vi "Rx Buffered Packet Page.vi"(8 "error in (no error)":errorcluster, 11 "Node Ptr":T4 format="%.0x") -> (0 "error out":errorcluster)   [LabVIEW 2016, in "UDP-Custom-Device System Explorer.lvlib"]
uses:
  UDP-Custom-Device System Explorer.lvlib
  Shared/Types/Shared - New Data Options.ctl
  Shared/Types/Shared - Receive Buffer Options.ctl
  Shared/Types/Shared - Pointer Encoding.ctl
  <vilib>/NI Veristand/Custom Device API/Custom Device Item Ref.ctl
  Types/Page References/Refs - Rx Buffered Data Packet Page.ctl
  <vilib>/NI VeriStand/Custom Device API/Custom Device API.lvlib
  Property Accessors/Shared Packet Accessors.lvlib
  Property Accessors/Buffered Data Packet.lvlib
  Property Accessors/Rx Packet Accessors.lvlib
  Shared/UDP-Custom-Device Shared.lvlib
panel:
  in  "Debug Mode":bool caption="Auto-Assign Local NIC"
  in  "Buffer Options":T1
  in  "New Data Options":T2
  in  "Pointer Encoding":T3
  in  "Multicast?":bool caption="Auto-Assign Local NIC"
  in  "Multicast IP Address":string
  in  "Read Timeout (ms)":i32
  in  "Prepend\nHeader?":bool caption="Auto-Assign Local NIC"
  in  "External Buffer?":bool
  in  "Buffer Size (bytes)":u32
  in  "Configure Header":bool
  in  "Endianness":u16(ring) items=["big-endian"=0, "little-endian"=2]
  in  "General Header 3":cluster{"Section Name":string}={"Section Name"="Network Settings"}
  out "Packet ID":i32
  in  "Auto-Assign Local NIC":bool
  in  "Port":u16
  in  "IP Address of Local NIC":string
  in  "Description":string
  in  "Name":string
  in  "General Header 2":cluster{"Section Name":string}={"Section Name"="Buffer Configuration"}
  in  "SHDocVw.IWebBrowser":refnum<k7>(container)
  in  "General Header":cluster{"Section Name":string}={"Section Name"="Packet Configuration"}
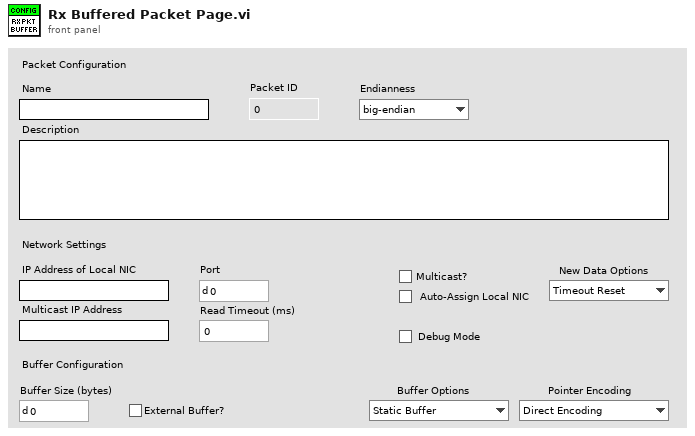
[diagram p1: front panel]
types:
  T1 = typedef "UDP-Custom-Device Shared.lvlib/Shared - Receive Buffer Options.ctl" = enum16{"Static Buffer", "Circular Buffer", "Circular Buffer + Size"}
  T2 = typedef "UDP-Custom-Device Shared.lvlib/Shared - New Data Options.ctl" = enum16{"Timeout Reset", "Counter"}
  T3 = typedef "UDP-Custom-Device Shared.lvlib/Shared - Pointer Encoding.ctl" = enum16{"Direct Encoding", "Conversion Encoding"}
  T4 = typedef "Custom Device API.lvlib/Custom Device Item Ref.ctl" = u64
  T5 = typedef "UDP-Custom-Device System Explorer.lvlib/Refs - Rx Buffered Data Packet Page.ctl" = cluster{"Name":refnum<vi>, "Description":refnum<vi>, "Packet ID":refnum<vi>, "Endianness":refnum<vi>, "Prepend\nHeader?":refnum<vi>, "Configure Header":refnum<vi>, "IP Address of Local NIC":refnum<vi>, "Port":refnum<vi>, "Auto-Assign Local NIC":refnum<vi>, "External Buffer?":refnum<vi>, "Buffer Size (bytes)":refnum<vi>, "Read Timeout (ms)":refnum<vi>, "Multicast?":refnum<vi>, "Multicast IP Address":refnum<vi>, "Pointer Encoding":refnum<vi>, "New Data Options":refnum<vi>, "Debug Mode":refnum<vi>, "Buffer Options":refnum<vi>}
  T6 = enum8{"Enabled", "Disabled", "Disabled and Grayed Out"}
  T7 = typedef "Custom Device API.lvlib/Custom Device Commands.ctl" = enum16{"Default", "Item renamed", "Shutdown", "Dynamic button pressed"}
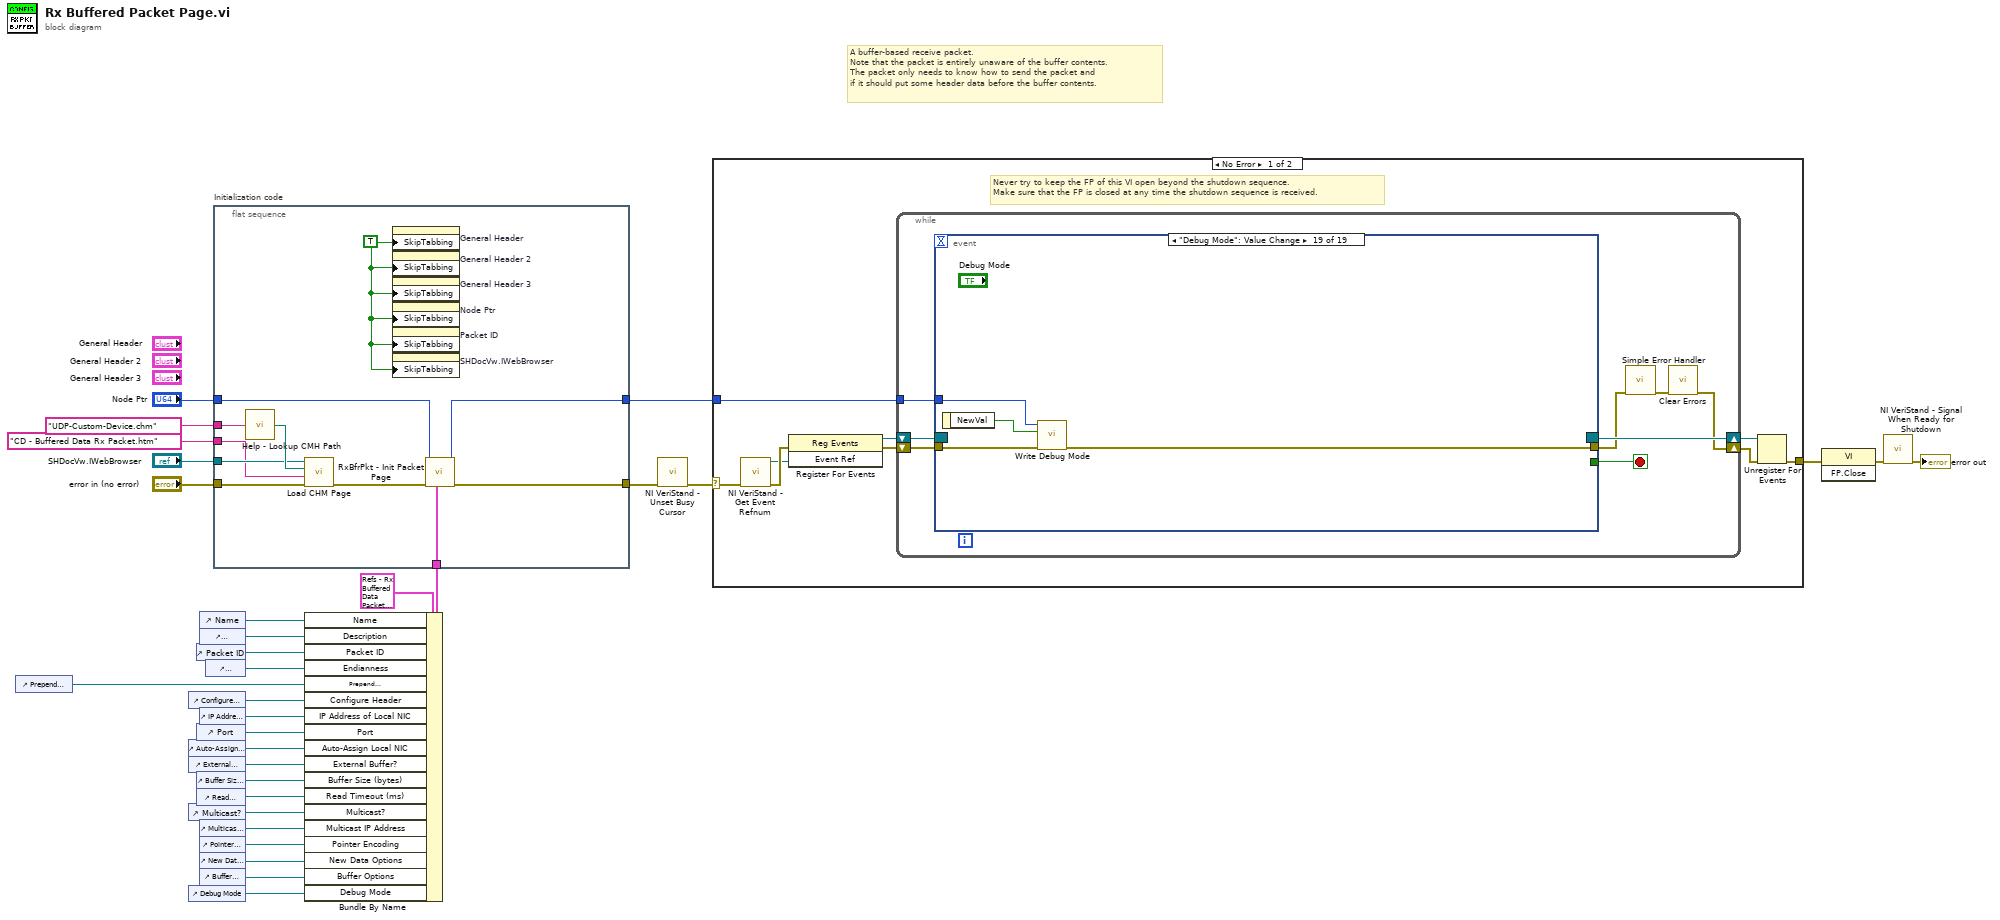
[diagram p0: block diagram]
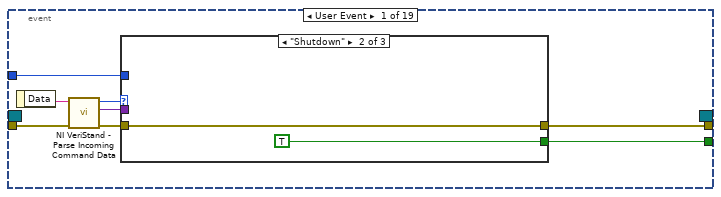
[diagram p2: hidden frame]
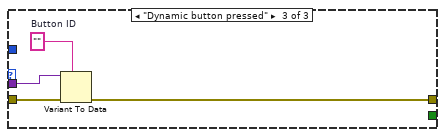
[diagram p4: hidden frame]
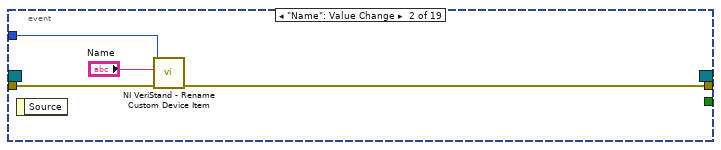
[diagram p5: hidden frame]
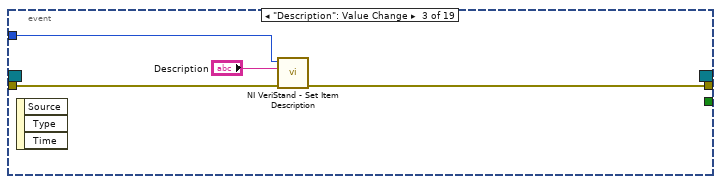
[diagram p6: hidden frame]
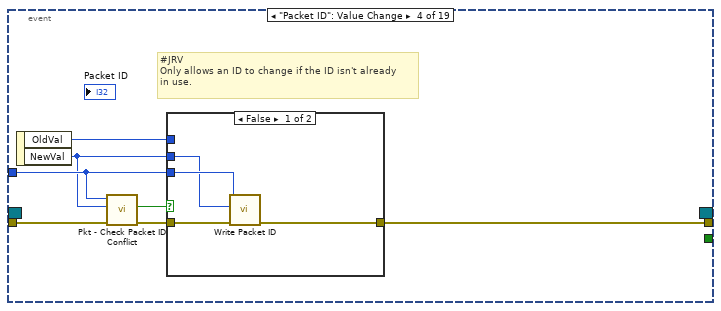
[diagram p7: hidden frame]
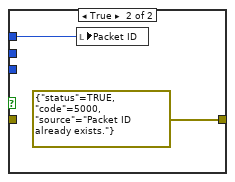
[diagram p8: hidden frame]
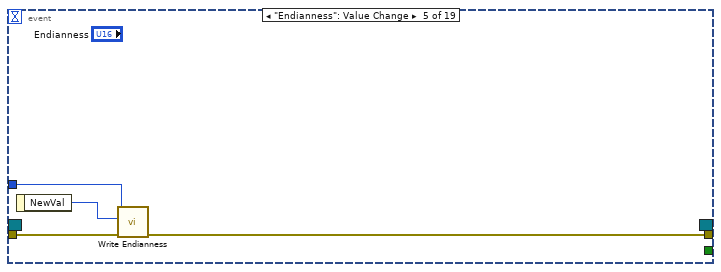
[diagram p9: hidden frame]
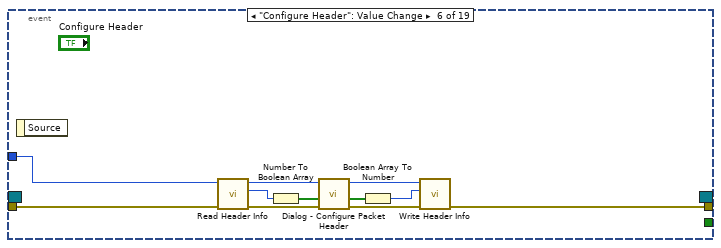
[diagram p10: hidden frame]
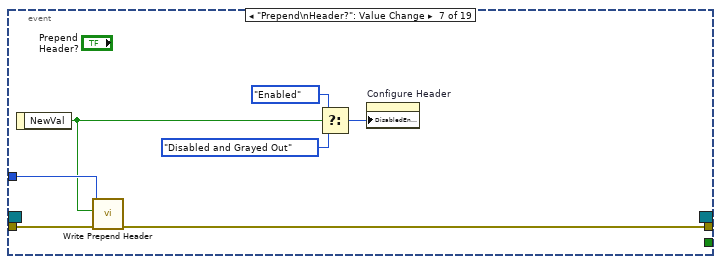
[diagram p11: hidden frame]
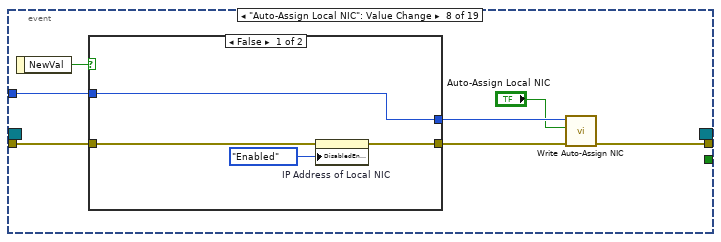
[diagram p12: hidden frame]
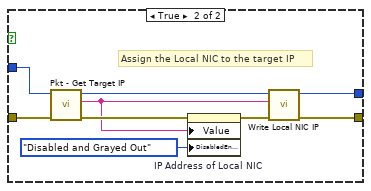
[diagram p13: hidden frame]
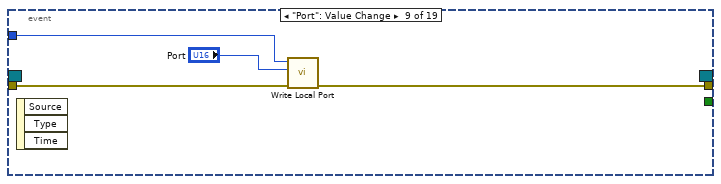
[diagram p14: hidden frame]
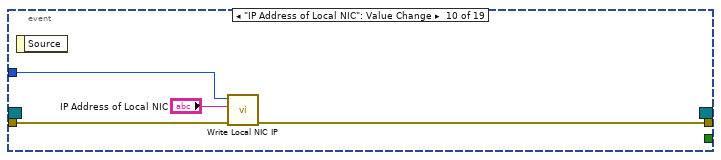
[diagram p15: hidden frame]
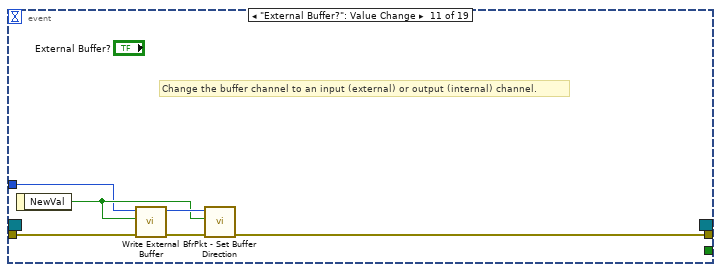
[diagram p16: hidden frame]
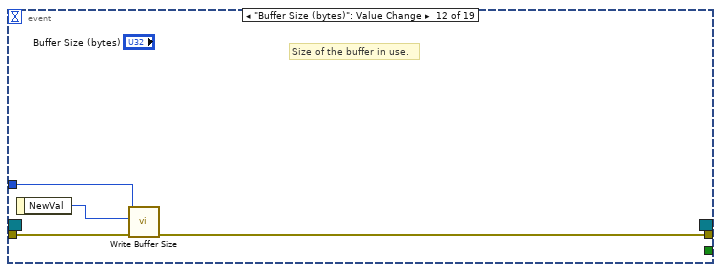
[diagram p17: hidden frame]
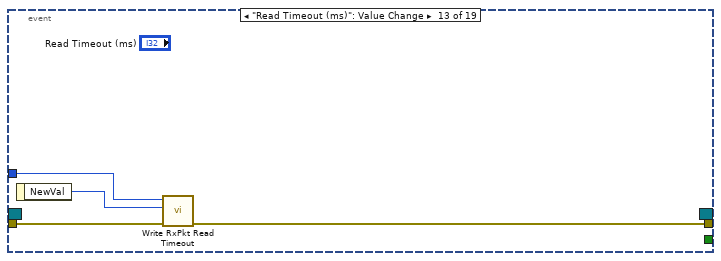
[diagram p18: hidden frame]
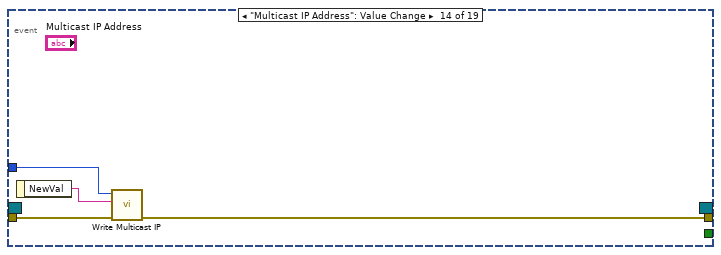
[diagram p19: hidden frame]
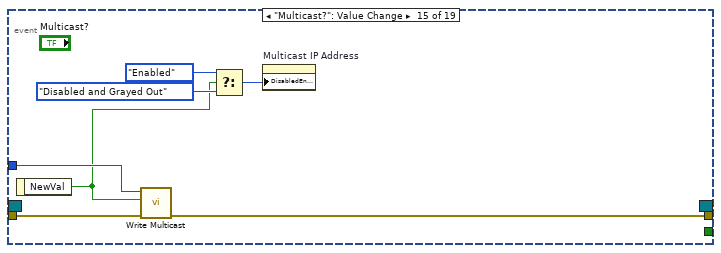
[diagram p20: hidden frame]
diagram:
  # "A buffer-based receive packet.\nNote that the packet is entirely unaware of the buffer contents.\nThe packet only needs to know how to send the packet and\nif it should put some header data before the buffer contents."
  n1 = control-ref of="Prepend\nHeader?"() -> (w14:refnum<vi>)
  n2 = control-ref of="Configure Header"() -> (w13:refnum<vi>)
  n3 = control-ref of="Auto-Assign Local NIC"() -> (w10:refnum<vi>)
  n4 = control-ref of="External Buffer?"() -> (w9:refnum<vi>)
  n5 = control-ref of="Multicast?"() -> (w6:refnum<vi>)
  n6 = control-ref of="Debug Mode"() -> (w2:refnum<vi>)
  n7 = control-ref of="Packet ID"() -> (w16:refnum<vi>)
  n8 = control-ref of="Port"() -> (w11:refnum<vi>)
  n9 = control-ref of="Buffer Size (bytes)"() -> (w8:refnum<vi>)
  n10 = control-ref of="Read Timeout (ms)"() -> (w7:refnum<vi>)
  n11 = control-ref of="Name"() -> (w18:refnum<vi>)
  n12 = control-ref of="Description"() -> (w17:refnum<vi>)
  n13 = control-ref of="IP Address of Local NIC"() -> (w12:refnum<vi>)
  n14 = control-ref of="Multicast IP Address"() -> (w5:refnum<vi>)
  n15 = control-ref of="Pointer Encoding"() -> (w4:refnum<vi>)
  n16 = control-ref of="New Data Options"() -> (w3:refnum<vi>)
  n17 = control-ref of="Buffer Options"() -> (w1:refnum<vi>)
  n18 = control-ref of="Endianness"() -> (w15:refnum<vi>)
  n19 = flat-sequence "Initialization code" {
    tunnel: "error in (no error)" -> [w41]
    tunnel: "Node Ptr" -> [w36]
    tunnel: [w33] -> w27
    tunnel: "SHDocVw.IWebBrowser" -> [w39]
    tunnel: "CD - Buffered Data Rx Packet.htm" ("CD_CHM_Section") -> [w38]
    tunnel: "UDP-Custom-Device.chm" ("CD_CHM_FileName") -> [w40]
    tunnel: [w35] -> w22
    tunnel: w19 -> [w32]
    frame #0 {
      w37 = TRUE ("Skip When Tabbing")
      n20 = call "Help - Lookup CMH Path.vi"("Main CMH File"=w40) -> ("Compiled CMH Path"=w42:path)
      n21 = call <vilib>:"Load CHM Page.vi"("error in (no error)"=w41, "HTML File"=w38, "Compiled CHM Path"=w42, "Web Browser Reference"=w39) -> ("error out"=w34:errorcluster)  [unwired: 7 in]
      n22 = property on="General Header" class="Clust (strict)"("SkipTabbing"=w37) -> ()  [unwired: 2 in, 2 out]
      n23 = property on="General Header 2" class="Clust (strict)"("SkipTabbing"=w37) -> ()  [unwired: 2 in, 2 out]
      n24 = property on="General Header 3" class="Clust (strict)"("SkipTabbing"=w37) -> ()  [unwired: 2 in, 2 out]
      n25 = property on="Node Ptr" class="DigNum (strict)"("SkipTabbing"=w37) -> ()  [unwired: 2 in, 2 out]
      n26 = property on="Packet ID" class="DigNum (strict)"("SkipTabbing"=w37) -> ()  [unwired: 2 in, 2 out]
      n27 = property on="SHDocVw.IWebBrowser" class="AXCont"("SkipTabbing"=w37) -> ()  [unwired: 2 in, 2 out]
      n28 = call "RxBfrPkt - Init Packet Page.vi"("Rx Buffered Data Packet Refs"=w32, "error in (no error)"=w34, "Node Ptr In"=w36) -> ("error out"=w33:errorcluster, "Node Ptr Out"=w35:T4)  [unwired: 7 in]
    }
  }
  n29 = Bundle By Name(cluster=T5 {"Name"=refnum, "Description"=refnum, "Packet ID"=refnum, "Endianness"=refnum, "Prepend\nHeader?"=refnum, "Configure Header"=refnum, "IP Address of Local NIC"=refnum, "Port"=refnum, "Auto-Assign Local NIC"=refnum, "External Buffer?"=refnum, "Buffer Size (bytes)"=refnum, "Read Timeout (ms)"=refnum, "Multicast?"=refnum, "Multicast IP Address"=refnum, "Pointer Encoding"=refnum, "New Data Options"=refnum, "Debug Mode"=refnum, "Buffer Options"=refnum} ("Rx Buffered Data Packet Refs"), "Name"=w18, "Description"=w17, "Packet ID"=w16, "Endianness"=w15, "Prepend\nHeader?"=w14, "Configure Header"=w13, "IP Address of Local NIC"=w12, "Port"=w11, "Auto-Assign Local NIC"=w10, "External Buffer?"=w9, "Buffer Size (bytes)"=w8, "Read Timeout (ms)"=w7, "Multicast?"=w6, "Multicast IP Address"=w5, "Pointer Encoding"=w4, "New Data Options"=w3, "Buffer Options"=w1, "Debug Mode"=w2) -> (w19:T5)
  n30 = call <vilib>:"NI VeriStand - Unset Busy Cursor.vi"("error in (no error)"=w27) -> ("error out"=w26:errorcluster)  [unwired: 10 out]
  n31 = case shown="No Error" w26 {
    selector: w26 -> [w43 w189]
    tunnel: [w48 w187] -> w31
    tunnel: w22 -> [w44 _]
    frame No Error {
      # "Never try to keep the FP of this VI open beyond the shutdown sequence.\nMake sure that the FP is closed at any time the shutdown sequence is received."
      n32 = call <vilib>:"NI VeriStand - Get Event Refnum.vi"("error in (no error)"=w43) -> ("error out"=w51:errorcluster, "Event Ref"=w47:refnum<user-event>)  [unwired: 9 out]
      n33 = register-events(error in=w51, w47) -> (reference out=w45:refnum<event-registration>, error out=w46:errorcluster)  [unwired: 1 in]
      n34 = while {
        tunnel: w44 -> [w55]
        shift-right: [w52] -> w49
        shift-left: w46 -> [w58]
        shift-right: [w59] -> w50
        shift-left: w45 -> [w57]
        stop <- w56 stop-if-true
        n35 = event shown="[18] \"Debug Mode\": Value Change" {
          selector: w57 -> [_ _ _ _ _ _ _ _ _ _ _ _ _ _ _ _ _ _ _]
          dyn-events: [_ _ _ _ _ _ _ _ _ _ _ _ _ _ _ _ _ _ _] -> w59
          timeout: _ -> [_ _ _ _ _ _ _ _ _ _ _ _ _ _ _ _ _ _ _]
          tunnel: w58 -> [w67 w78 w82 w87 w98 w107 w114 w124 w140 w145 w147 w153 w157 w161 w169 w173 w176 w182 w184]
          tunnel: [w63 _ _ _ _ _ _ _ _ _ _ _ _ _ _ _ _ _ _] -> w56
          tunnel: [w62 w76 w79 w89 w97 w101 w111 w119 w139 w144 w146 w152 w156 w160 w168 w171 w175 w179 w183] -> w54
          tunnel: w55 -> [w61 w77 w81 w88 w99 w108 w115 w123 w141 w142 w148 w155 w159 w163 w170 w174 w178 w181 w186]
          event User Event {
            n36 = event-data() -> ("Data"=w66:string)  [unwired: 1 out]
            n37 = call <vilib>:"NI VeriStand - Parse Incoming Command Data.vi"("error in (no error)"=w67, "Incoming data"=w66) -> ("error out"=w65:errorcluster, "Outgoing data"=w60:variant, "Action"=w64:T7)  [unwired: 7 out]
            n38 = case shown="\"Shutdown\"" w64 {
              tunnel: w65 -> [w68 w69 w74]
              tunnel: [_ TRUE _] -> w63
              tunnel: [w68 w69 w71] -> w62
              tunnel: w61 -> [_ _ _]
              tunnel: w60 -> [_ _ w73]
              frame "Default", Default {
              }
              frame "Shutdown" {
              }
              frame "Dynamic button pressed" {
                w72 = ""  # Button ID
                n39 = Variant To Data(error in=w74, type=w72, Variant=w73) -> (error out=w71:errorcluster)  [unwired: 1 out]
              }
            }
          }
          event "Name": Value Change {
            n40 = event-data() -> ()  [unwired: 2 out]
            n41 = call <vilib>:"NI VeriStand - Rename Custom Device Item.vi"("error in (no error)"=w78, "New Name"="Name", "Item Ref in"=w77) -> ("error out"=w76:errorcluster)  [unwired: 6 in, 2 out]
          }
          event "Description": Value Change {
            n42 = event-data() -> ()  [unwired: 4 out]
            n43 = call <vilib>:"NI VeriStand - Set Item Description.vi"("error in (no error)"=w82, "Description"="Description", "Item Ref in"=w81) -> ("error out"=w79:errorcluster)  [unwired: 6 in, 2 out]
          }
          event "Packet ID": Value Change {
            # "#JRV\nOnly allows an ID to change if the ID isn't already\nin use."
            n44 = event-data() -> ("OldVal"=w83:i32, "NewVal"=w84:i32)  [unwired: 1 out]
            n45 = call "Pkt - Check Packet ID Conflict.vi"("error in (no error)"=w87, "New ID"=w84, "Packet Ref In"=w88) -> ("error out"=w86:errorcluster, "Conflicting ID?"=w85:bool)  [unwired: 7 in]
            n46 = case shown="False" w85 {
              tunnel: [w92 errorcluster {"status"=TRUE, "code"=5000, "source"="Packet ID already exists."} ("error out")] -> w89
              tunnel: w88 -> [w91 _]
              tunnel: w86 -> [w93 _]
              tunnel: w84 -> [w90 _]
              tunnel: w83 -> [_ w95]
              frame False {
                n47 = call "Write Packet ID.vi"("error in (no error)"=w93, "Packet ID"=w90, "Node Ptr"=w91) -> ("error out"=w92:errorcluster)  [unwired: 7 in, 1 out]
              }
              frame True {
                n48 = local write "Packet ID"(w95) -> ()
              }
            }
          }
          event "Endianness": Value Change {
            n49 = event-data() -> ("NewVal"=w96:u16)  [unwired: 1 out]
            n50 = call "Write Endianness.vi"("error in (no error)"=w98, "Endianness"=w96, "Node Ptr"=w99) -> ("error out"=w97:errorcluster)  [unwired: 7 in, 1 out]
          }
          event "Configure Header": Value Change {
            n51 = event-data() -> ()  [unwired: 2 out]
            n52 = call "Read Header Info.vi"("error in (no error)"=w107, "Node Ptr"=w108) -> ("error out"=w106:errorcluster, "Header Info"=w105:u32, "Node Ptr out"=w104:T4)  [unwired: 7 in]
            n53 = Number To Boolean Array(number=w105) -> (Boolean array=w110:bool[])
            n54 = call "Dialog - Configure Packet Header.vi"("error in (no error)"=w106, "Header Elements In"=w110, "Packet Ref in"=w104) -> ("error out"=w102:errorcluster, "Header Elements Out"=w109:bool[], "Packet Ref out"=w103:T4)  [unwired: 6 in]
            n55 = Boolean Array To Number(Boolean array=w109) -> (number=w100:u32)
            n56 = call "Write Header Info.vi"("error in (no error)"=w102, "Header Info"=w100, "Node Ptr"=w103) -> ("error out"=w101:errorcluster)  [unwired: 7 in, 1 out]
          }
          event "Prepend\nHeader?": Value Change {
            n57 = event-data() -> ("NewVal"=w113:bool)  [unwired: 1 out]
            n58 = call "Write Prepend Header.vi"("error in (no error)"=w114, "Prepend Header"=w113, "Node Ptr"=w115) -> ("error out"=w111:errorcluster)  [unwired: 7 in, 1 out]
            n59 = Select(t=T6."Enabled" ("Disabled"), s=w113, f=T6."Disabled and Grayed Out" ("Disabled")) -> (s? t:f=w112:T6)
            n60 = property on="Configure Header" class="Bool"("DisabledEnum"=w112) -> ()  [unwired: 2 in, 2 out]
          }
          event "Auto-Assign Local NIC": Value Change {
            n61 = event-data() -> ("NewVal"=w122:bool)  [unwired: 1 out]
            n62 = case shown="False" w122 {
              tunnel: w123 -> [w126 w136]
              tunnel: w124 -> [w127 w137]
              tunnel: [w128 w129] -> w120
              tunnel: [w126 w132] -> w121
              frame False {
                n63 = property on="IP Address of Local NIC" class="Str"(error in=w127, "DisabledEnum"=T6."Enabled" ("Disabled")) -> (error out=w128:errorcluster)  [unwired: 1 in, 1 out]
              }
              frame True {
                # "Assign the Local NIC to the target IP"
                n64 = call "Pkt - Get Target IP.vi"("error in"=w137, "Item Ref in"=w136) -> ("error out"=w135:errorcluster, "IPAddress"=w131:string, "Item Ref out"=w133:T4)  [unwired: 7 in]
                n65 = property on="IP Address of Local NIC" class="Str"(error in=w135, "Value"=w131, "DisabledEnum"=T6."Disabled and Grayed Out" ("Disabled")) -> (error out=w130:errorcluster)  [unwired: 1 in, 1 out]
                n66 = call "Write Local NIC IP.vi"("error in (no error)"=w130, "IP Address of Local NIC"=w131, "Node Ptr"=w133) -> ("error out"=w129:errorcluster, "Node Ptr out"=w132:T4)  [unwired: 7 in]
              }
            }
            n67 = call "Write Auto-Assign NIC.vi"("error in (no error)"=w120, "Auto-Assign NIC"="Auto-Assign Local NIC", "Node Ptr"=w121) -> ("error out"=w119:errorcluster)  [unwired: 7 in, 1 out]
          }
          event "Port": Value Change {
            n68 = event-data() -> ()  [unwired: 4 out]
            n69 = call "Write Local Port.vi"("error in (no error)"=w140, "Port"="Port", "Node Ptr"=w141) -> ("error out"=w139:errorcluster)  [unwired: 7 in, 1 out]
          }
          event "IP Address of Local NIC": Value Change {
            n70 = event-data() -> ()  [unwired: 2 out]
            n71 = call "Write Local NIC IP.vi"("error in (no error)"=w145, "IP Address of Local NIC"="IP Address of Local NIC", "Node Ptr"=w142) -> ("error out"=w144:errorcluster)  [unwired: 7 in, 1 out]
          }
          event "External Buffer?": Value Change {
            # "Change the buffer channel to an input (external) or output (internal) channel."
            n72 = event-data() -> ("NewVal"=w149:bool)  [unwired: 1 out]
            n73 = call "Write External Buffer.vi"("error in (no error)"=w147, "External Buffer"=w149, "Node Ptr"=w148) -> ("error out"=w151:errorcluster, "Node Ptr out"=w150:T4)  [unwired: 7 in]
            n74 = call "BfrPkt - Set Buffer Direction.vi"("error in (no error)"=w151, "External?"=w149, "Node Ptr"=w150) -> ("error out"=w146:errorcluster)  [unwired: 7 in, 1 out]
          }
          event "Buffer Size (bytes)": Value Change {
            # "Size of the buffer in use."
            n75 = event-data() -> ("NewVal"=w154:u32)  [unwired: 1 out]
            n76 = call "Write Buffer Size.vi"("error in (no error)"=w153, "Buffer Size"=w154, "Node Ptr"=w155) -> ("error out"=w152:errorcluster)  [unwired: 7 in, 1 out]
          }
          event "Read Timeout (ms)": Value Change {
            n77 = event-data() -> ("NewVal"=w158:i32)  [unwired: 1 out]
            n78 = call "Write RxPkt Read Timeout.vi"("error in (no error)"=w157, "Read Timeout"=w158, "Node Ptr"=w159) -> ("error out"=w156:errorcluster)  [unwired: 7 in, 1 out]
          }
          event "Multicast IP Address": Value Change {
            n79 = event-data() -> ("NewVal"=w162:string)  [unwired: 1 out]
            n80 = call "Write Multicast IP.vi"("error in (no error)"=w161, "Multicast IP Address"=w162, "Node Ptr"=w163) -> ("error out"=w160:errorcluster)  [unwired: 7 in, 1 out]
          }
          event "Multicast?": Value Change {
            n81 = event-data() -> ("NewVal"=w165:bool)  [unwired: 1 out]
            n82 = call "Write Multicast.vi"("error in (no error)"=w169, "Multicast"=w165, "Node Ptr"=w170) -> ("error out"=w168:errorcluster)  [unwired: 7 in, 1 out]
            n83 = Select(t=T6."Enabled" ("Disabled"), s=w165, f=T6."Disabled and Grayed Out" ("Disabled")) -> (s? t:f=w164:T6)
            n84 = property on="Multicast IP Address" class="Str"("DisabledEnum"=w164) -> ()  [unwired: 2 in, 2 out]
          }
          event Value Change {
            n85 = event-data() -> ("NewVal"=w172:T3)  [unwired: 1 out]
            n86 = call "Write Pointer Encoding.vi"("error in (no error)"=w173, "Pointer Encoding"=w172, "Node Ptr"=w174) -> ("error out"=w171:errorcluster)  [unwired: 7 in, 1 out]
          }
          event Value Change {
            n87 = event-data() -> ("NewVal"=w177:T2)  [unwired: 1 out]
            n88 = call "Write RxPkt New Data Option.vi"("error in (no error)"=w176, "New Data Option"=w177, "Node Ptr"=w178) -> ("error out"=w175:errorcluster)  [unwired: 7 in, 1 out]
          }
          event Value Change {
            n89 = event-data() -> ("NewVal"=w180:T1)  [unwired: 1 out]
            n90 = call "Write Rx Buffer Option.vi"("error in (no error)"=w182, "Buffer Option"=w180, "Node Ptr"=w181) -> ("error out"=w179:errorcluster)  [unwired: 7 in, 1 out]
          }
          event "Debug Mode": Value Change {
            n91 = event-data() -> ("NewVal"=w185:bool)  [unwired: 1 out]
            n92 = call "Write Debug Mode.vi"("error in (no error)"=w184, "Debug Mode"=w185, "Node Ptr"=w186) -> ("error out"=w183:errorcluster)  [unwired: 7 in, 1 out]
          }
        }
        n93 = call <vilib>:"Simple Error Handler.vi"("error in (no error)"=w54) -> ("error out"=w53:errorcluster)  [unwired: 1 in, 7 out]
        n94 = call <vilib>:"Clear Errors.vi"("error in (no error)"=w53) -> ("error out"=w52:errorcluster)  [unwired: 1 in, 5 out]
      }
      n95 = Unregister For Events(event registration refnum=w50, error in=w49) -> (error out=w48:errorcluster)
    }
    frame Error {
      n96 = call <vilib>:"Simple Error Handler.vi"("error in (no error)"=w189) -> ("error out"=w188:errorcluster)  [unwired: 1 in, 7 out]
      n97 = call <vilib>:"Clear Errors.vi"("error in (no error)"=w188) -> ("error out"=w187:errorcluster)  [unwired: 1 in, 5 out]
    }
  }
  n98 = invoke class="VI" method="FP.Close"(error in=w31) -> (error out=w30:errorcluster)  [unwired: 2 in, 2 out]
  n99 = call <vilib>:"NI VeriStand - Signal When Ready for Shutdown.vi"("error in (no error)"=w30) -> ("error out"=→"error out":errorcluster)  [unwired: 10 out]
